vi "PV HiScroll Control commands .vi"(8 "error in (no error)":errorcluster, 9 "PV HiScroll Control commands - Cluster":T1={"Parameter"=enum."Standby [002]", "Parameter\nread only<->describe"=FALSE, "off        on"=TRUE, "Control via interface"=1, "Configuration DO2 / DO1"=5, "Configuration input DI2"=0} caption="Operating adjustment - Cluster" {"Configuration input DI2" items=["0 = deactivated", "1 = deactivated", "2 = deactivated", "3 = deactivated", "4 = deactivated", "5 = Speed actuator operation on"]; "Control via interface" items=["remote"=1, "RS 485"=2, "Unlock the interface selection"=255]; "Configuration DO2 / DO1" items=["1 = no error"=1, "2 = error"=2, "5 = target speed is reached"=5, "6 = pump on"=6, "9 = always \"0\""=9, "10 = always \"1\""=10, "11 = remote priority active"=11, "21 = gas ballast"=21]}, 10 "Adress of unit":u16=1 min=1 max=999 step=1, 11 "VISA session":refnum<visa-resource-name>) -> (0 "error out":errorcluster, 2 "response (data)":string, 3 "dup VISA session":refnum<visa-resource-name>)   [LabVIEW 2021, in "Pfeiffer Vacuum.lvlib"]
doc: "There are 15 parameters available, only one of which can be enabled at a time. \n\nStandby [002]\nAuto-Standby [006]\nFault acknowledgment [009]\nPump [010]\nAuto-Boost [011]\nConfiguration output DO2 [019]\nPressure mode [020]\nConfiguration output DO1 [024]\nSpeed setting mode [026]\nAuto-Start [034]\nGas ballast valve control [052]\nControl via interface [060]\nInterface selection locked [061]\nConfiguration DI2 [063]\nFactory settings [095]\n\nNote: The controls right of this one will set the appropriate values for the selected parameter. Any settings for an parameter that is not selected will be ignored. If a value is out of range, it will be changed to either the upper or the lower limit of the range."
uses:
  <instrlib>/Pfeiffer Vacuum/Pfeiffer Vacuum.lvlib
  <instrlib>/Pfeiffer Vacuum/Public/HiScroll/PV HiScroll Control commands - Cluster.ctl
panel:
  # "Standby                                   \n Auto standby\n Pump \n Auto boost\n Pressure mode\n Speed setting mode \n Auto start\n Gas ballast valve control \n Interface selection locked"
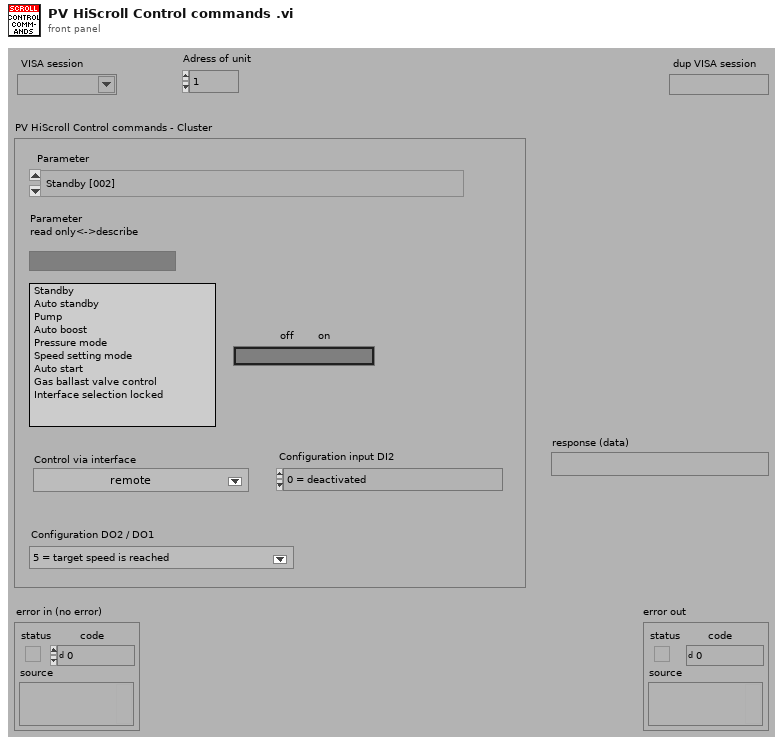
[diagram p1: front panel]
types:
  T1 = typedef "Pfeiffer Vacuum.lvlib/PV HiScroll Control commands - Cluster.ctl" = cluster{"Parameter":enum16{"Standby [002]", "Auto-Standby [006]", "Fault acknowledgment [009]", "Pump [010]", "Auto-Boost [011]", "Configuration output DO2 [019]", "Pressure mode [020]", "Configuration output DO1 [024]", "Speed setting mode [026]", "Auto-Start [034]", "Gas ballast valve control [052]", "Control via interface [060]", "Interface selection locked [061]", "Configuration input DI2 [063]", "Factory Settings [095]"}, "Parameter\nread only<->describe":bool, "off        on":bool, "Control via interface":u16, "Configuration DO2 / DO1":u16, "Configuration input DI2":u16}
  T2 = enum16{"Standby [002]", "Auto-Standby [006]", "Fault acknowledgment [009]", "Pump [010]", "Auto-Boost [011]", "Configuration output DO2 [019]", "Pressure mode [020]", "Configuration output DO1 [024]", "Speed setting mode [026]", "Auto-Start [034]", "Gas ballast valve control [052]", "Control via interface [060]", "Interface selection locked [061]", "Configuration input DI2 [063]", "Factory Settings [095]"}
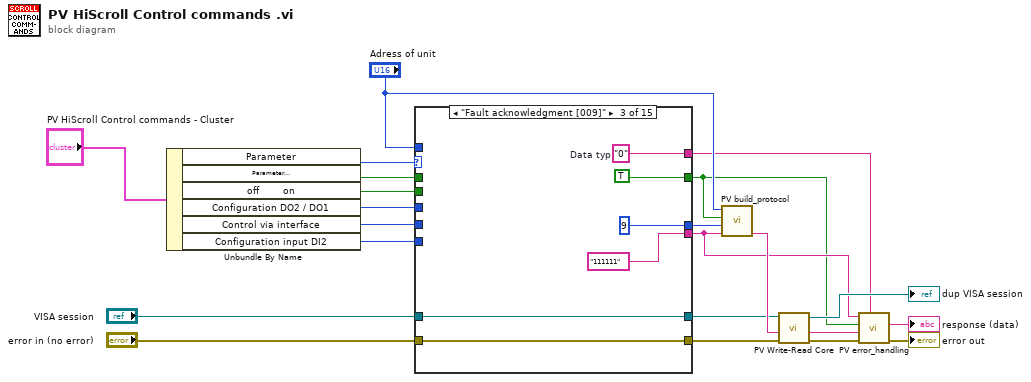
[diagram p0: block diagram]
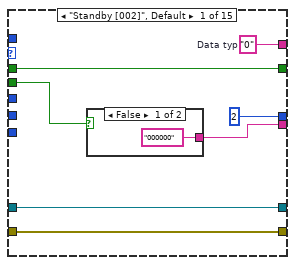
[diagram p2: hidden frame]
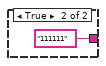
[diagram p3: hidden frame]
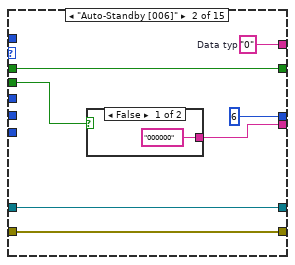
[diagram p4: hidden frame]
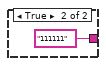
[diagram p5: hidden frame]
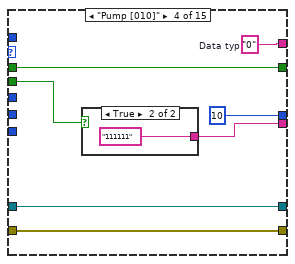
[diagram p6: hidden frame]
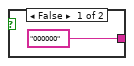
[diagram p7: hidden frame]
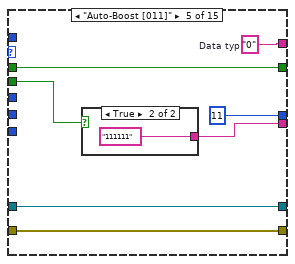
[diagram p8: hidden frame]
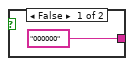
[diagram p9: hidden frame]
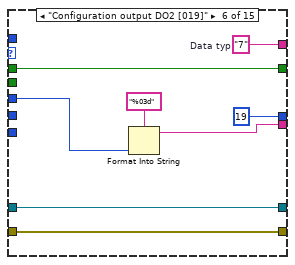
[diagram p10: hidden frame]
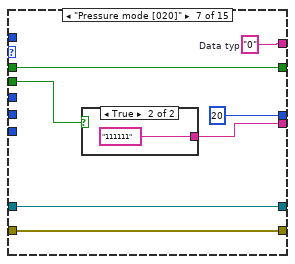
[diagram p11: hidden frame]
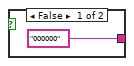
[diagram p12: hidden frame]
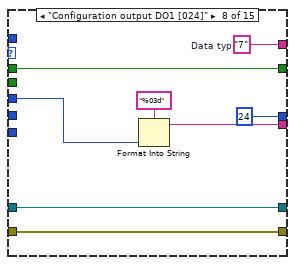
[diagram p13: hidden frame]
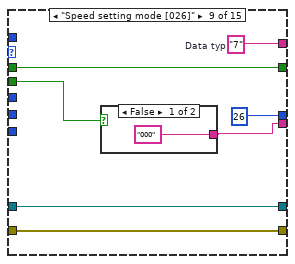
[diagram p14: hidden frame]
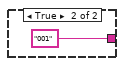
[diagram p15: hidden frame]
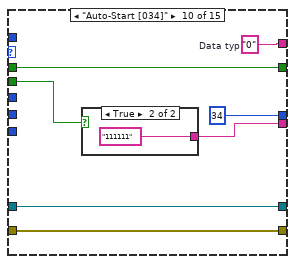
[diagram p16: hidden frame]
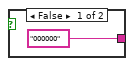
[diagram p17: hidden frame]
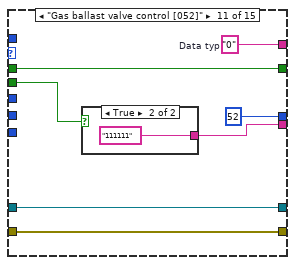
[diagram p18: hidden frame]
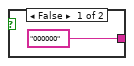
[diagram p19: hidden frame]
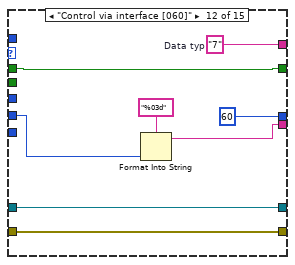
[diagram p20: hidden frame]
diagram:
  n1 = Unbundle By Name("PV HiScroll Control commands - Cluster") -> ("Parameter"=w21:T2, "Parameter\nread only<->describe"=w20:bool, "off        on"=w5:bool, "Configuration DO2 / DO1"=w4:u16, "Control via interface"=w3:u16, "Configuration input DI2"=w2:u16)
  n2 = case shown="\"Fault acknowledgment [009]\"" w21 {
    tunnel: [u16 2 ("Parameter-number") u16 6 ("Parameter-number") u16 9 ("Parameter-number") u16 10 ("Parameter-number") u16 11 ("Parameter-number") u16 19 ("Parameter-number") u16 20 ("Parameter-number") u16 24 ("Parameter-number") u16 26 ("Parameter-number") u16 34 ("Parameter-number") u16 52 ("Parameter-number") u16 60 ("Parameter-number") u16 61 ("Parameter-number") u16 63 ("Parameter-number") u16 95 ("Parameter-number")] -> w22
    tunnel: [w28 w37 "111111" ("Data") w52 w61 w66 w78 w83 w92 w104 w108 w118 w127 w137 "111111" ("Data")] -> w10
    tunnel: [w27 w36 TRUE w51 w60 w72 w77 w88 w95 w103 w110 w121 w126 w139 w142] -> w8
    tunnel: w20 -> [w27 w36 _ w51 w60 w72 w77 w88 w95 w103 w110 w121 w126 w139 w142]
    tunnel: w5 -> [w26 w35 _ w50 w59 _ w76 _ w94 w102 w109 _ w125 _ _]
    tunnel: [w25 w34 w44 w49 w58 w71 w75 w87 w96 w101 w112 w120 w129 w140 w145] -> w9
    tunnel: "VISA session" -> [w24 w33 w43 w48 w57 w70 w74 w86 w91 w100 w114 w124 w131 w136 w144]
    tunnel: [w24 w33 w43 w48 w57 w70 w74 w86 w91 w100 w114 w124 w131 w136 w144] -> w15
    tunnel: "Adress of unit" -> [_ _ _ _ _ _ _ _ _ _ _ _ _ _ _]
    tunnel: "error in (no error)" -> [w23 w32 w42 w47 w56 w69 w73 w85 w90 w99 w113 w123 w130 w135 w143]
    tunnel: [w23 w32 w42 w47 w56 w69 w73 w85 w90 w99 w113 w123 w130 w135 w143] -> w14
    tunnel: w4 -> [_ _ _ _ _ w65 _ w82 _ _ _ _ _ _ _]
    tunnel: w3 -> [_ _ _ _ _ _ _ _ _ _ _ w117 _ _ _]
    tunnel: w2 -> [_ _ _ _ _ _ _ _ _ _ _ _ _ w134 _]
    frame "Standby [002]", Default {
      w25 = "0"  # Data typ
      n3 = case shown="False" w26 {
        tunnel: ["000000" ("Data") "111111" ("Data")] -> w28
        frame False {
        }
        frame True {
        }
      }
    }
    frame "Auto-Standby [006]" {
      w34 = "0"  # Data typ
      n4 = case shown="False" w35 {
        tunnel: ["000000" ("Data") "111111" ("Data")] -> w37
        frame False {
        }
        frame True {
        }
      }
    }
    frame "Fault acknowledgment [009]" {
      w44 = "0"  # Data typ
    }
    frame "Pump [010]" {
      w49 = "0"  # Data typ
      n5 = case shown="True" w50 {
        tunnel: ["000000" ("Data") "111111" ("Data")] -> w52
        frame False {
        }
        frame True {
        }
      }
    }
    frame "Auto-Boost [011]" {
      w58 = "0"  # Data typ
      n6 = case shown="True" w59 {
        tunnel: ["000000" ("Data") "111111" ("Data")] -> w61
        frame False {
        }
        frame True {
        }
      }
    }
    frame "Configuration output DO2 [019]" {
      w71 = "7"  # Data typ
      n7 = Format Into String(format string="%03d" ("Format-String"), w65) -> (resulting string=w66:string)  [unwired: 2 in, 1 out]
    }
    frame "Pressure mode [020]" {
      w75 = "0"  # Data typ
      n8 = case shown="True" w76 {
        tunnel: ["000000" ("Data") "111111" ("Data")] -> w78
        frame False {
        }
        frame True {
        }
      }
    }
    frame "Configuration output DO1 [024]" {
      w87 = "7"  # Data typ
      n9 = Format Into String(format string="%03d" ("Format-String"), w82) -> (resulting string=w83:string)  [unwired: 2 in, 1 out]
    }
    frame "Speed setting mode [026]" {
      w96 = "7"  # Data typ
      n10 = case shown="False" w94 {
        tunnel: ["000" ("Data") "001" ("Data")] -> w92
        frame False {
        }
        frame True {
        }
      }
    }
    frame "Auto-Start [034]" {
      w101 = "0"  # Data typ
      n11 = case shown="True" w102 {
        tunnel: ["000000" ("Data") "111111" ("Data")] -> w104
        frame False {
        }
        frame True {
        }
      }
    }
    frame "Gas ballast valve control [052]" {
      w112 = "0"  # Data typ
      n12 = case shown="True" w109 {
        tunnel: ["000000" ("Data") "111111" ("Data")] -> w108
        frame False {
        }
        frame True {
        }
      }
    }
    frame "Control via interface [060]" {
      w120 = "7"  # Data typ
      n13 = Format Into String(format string="%03d" ("Format-String"), w117) -> (resulting string=w118:string)  [unwired: 2 in, 1 out]
    }
    frame "Interface selection locked [061]" {
      w129 = "0"  # Data typ
      n14 = case shown="True" w125 {
        tunnel: ["000000" ("Data") "111111" ("Data")] -> w127
        frame False {
        }
        frame True {
        }
      }
    }
    frame "Configuration input DI2 [063]" {
      w140 = "7"  # Data typ
      n15 = Format Into String(format string="%03d" ("Format-String"), w134) -> (resulting string=w137:string)  [unwired: 2 in, 1 out]
    }
    frame "Factory Settings [095]" {
      w145 = "0"  # Data typ
    }
  }
  n16 = call <instrlib>:"PV build_protocol.vi"("Data"=w10, "Parameter-number"=w22, "parameter\nread<->describe"=w8, "Adress"="Adress of unit") -> ("output"=w16:string)  [unwired: 3 in]
  n17 = call <instrlib>:"PV Write-Read Core.vi"("error in"=w14, "Write data in"=w16, "VISA session"=w15) -> ("error out"=w12:errorcluster, "response (data) out"=w13:string, "dup VISA session"=→"dup VISA session":refnum<visa-resource-name>)  [unwired: 2 in]
  n18 = call <instrlib>:"PV error_handling.vi"("Data Typ in"=w9, "error in"=w12, "response (data) in"=w13, "Parameter\nread only<->describe"=w8, "data in"=w10) -> ("error out"=→"error out":errorcluster, "Data out"=→"response (data)":string)  [unwired: 4 in, 1 out]
